vi "walker_tester.vi"() -> ()   [LabVIEW 2010]
uses:
  <userlib>/Nanonis Prog Interface V5/Nanonis Prog Interface.lvlib
panel:
  in  "?":bool
  out "Delta":cluster{"index":i32, sgl}[](graph)
  out "Walk Halt":bool
  out "Walk Done":bool
  in  "Stop Walker":bool
  in  "Stop Loop":bool
  in  "Number of Steps":u16=500
  in  "Capacitance Limit":sgl=700.0
  out "Capacitance":cluster{"index":i32, sgl}[](graph)
  in  "?":bool
  in  "Frequency (Hz)":sgl=250.0
  in  "Amplitude (V)":sgl=150.0
  # "+Z"
  # "-Z"
  # "Absolute Value"
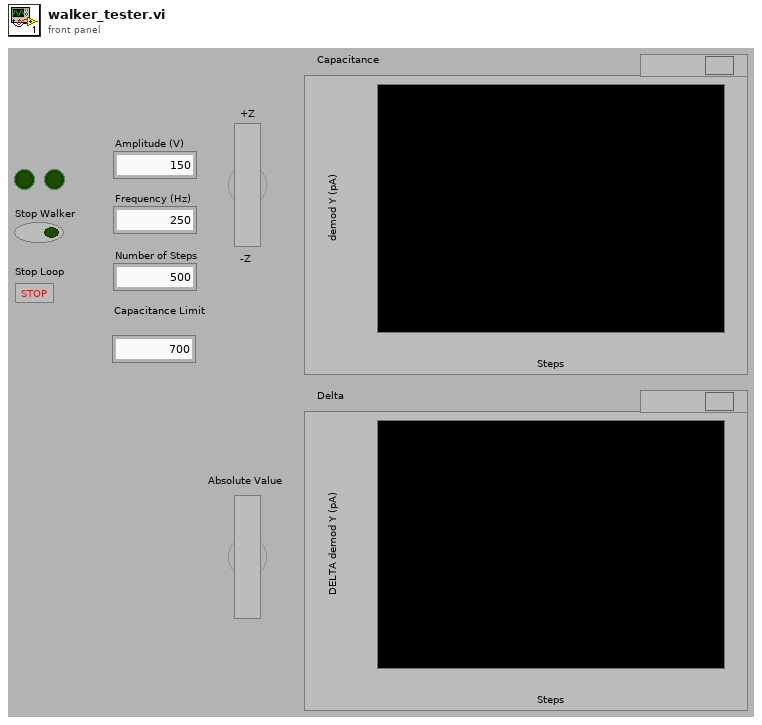
[diagram p1: front panel]
types:
  T1 = enum8{"Group 1", "Group 2", "Group 3", "Group 4", "Group 5", "Group 6"}
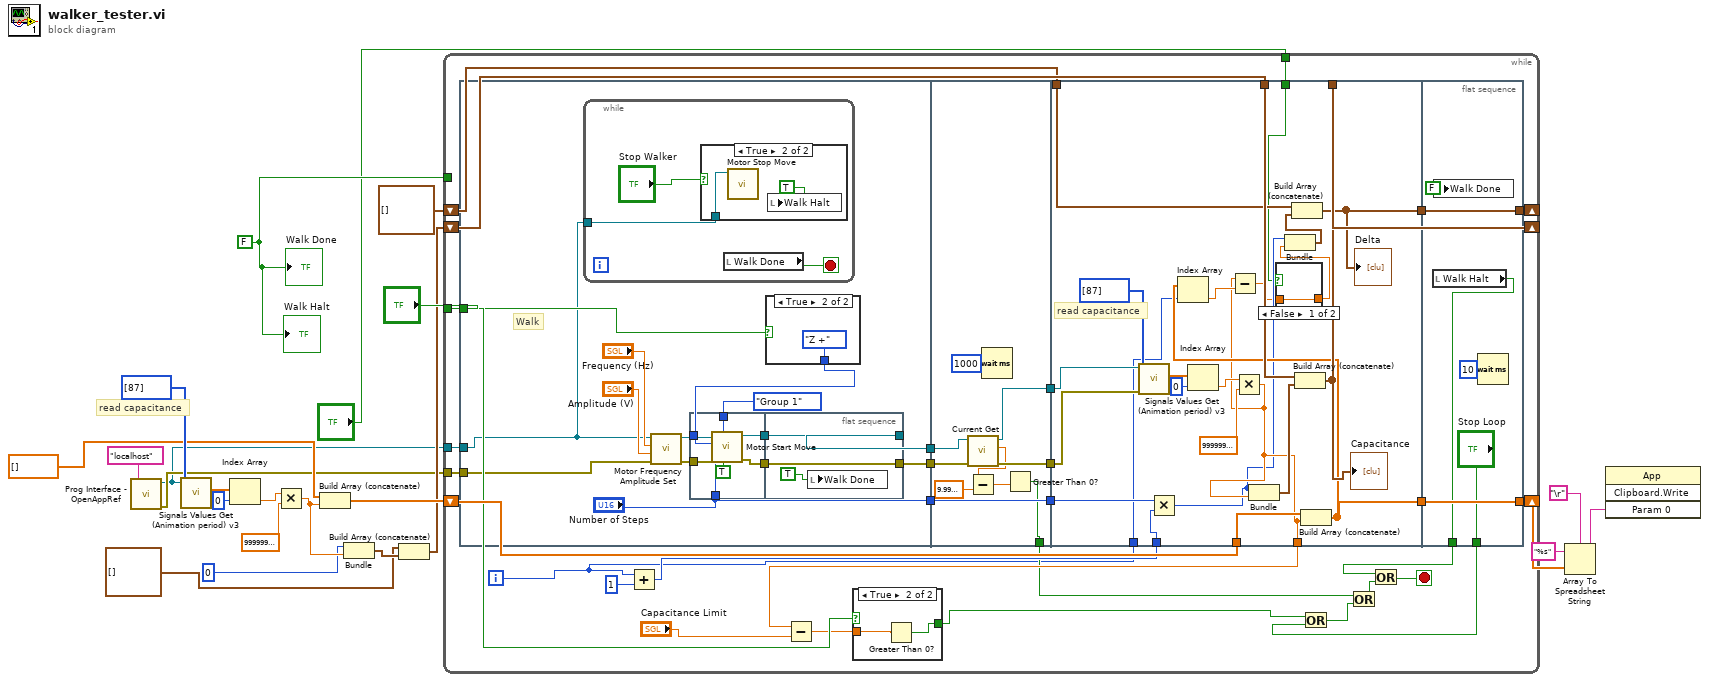
[diagram p0: block diagram]
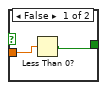
[diagram p2: hidden frame]
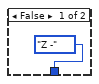
[diagram p4: hidden frame]
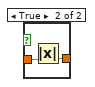
[diagram p5: hidden frame]
diagram:
  w3 = FALSE
  # "read capacitance"
  n1 = call <userlib>:"Prog Interface - OpenAppRef.vi"("Machine name (local machine IP)"="localhost" ("machine name (localhost)")) -> ("Error out"=w5:errorcluster, "Application reference"=w4:refnum<vi>)  [unwired: 5 in]
  n2 = call <userlib>:"Signals Values Get (Animation period) v3.vi"("Signals indexes (0-127)"=i8[] [87], "Application ref in"=w4) -> ("Signals Values"=w15:sgl[])  [unwired: 6 in, 2 out]
  n3 = Index Array(array=w15, index=0) -> (element=w14:sgl)
  n4 = Multiply(x=w14, y=sgl 1000000000000.0) -> (x*y=w10:sgl)
  n5 = Build Array (concatenate)(sgl[] [], w10) -> (w11:sgl[])
  n6 = Bundle("index"=0, w10) -> (w8:cluster{"index":i32, sgl})  [unwired: 1 in]
  n7 = Build Array (concatenate)(cluster{i32, sgl}[] [], w8) -> (w7:cluster{"index":i32, sgl}[])
  n8 = while {
    shift-right: [w52] -> _
    shift-left: w7 -> [w51]
    shift-right: [w50] -> w23
    shift-left: w11 -> [w49]
    tunnel: "?" -> [w47]
    tunnel: w4 -> [w39]
    tunnel: w5 -> [w38]
    tunnel: w3 -> [_]
    shift-right: [w26] -> _
    shift-left: cluster{i32, sgl}[] [] -> [w25]
    tunnel: "?" -> [w24]
    i -> [w28]
    stop <- w31 stop-if-true
    n9 = flat-sequence {
      tunnel: ["Number of Steps"] -> w54
      tunnel: w47 -> [w66]
      tunnel: w39 -> [w61]
      tunnel: w38 -> [w64]
      tunnel: [w63] -> w37
      tunnel: [w62] -> w36
      tunnel: w54 -> [w99]
      tunnel: [w99] -> w53
      tunnel: w37 -> [w98]
      tunnel: w36 -> [w97]
      tunnel: [w96] -> w35
      tunnel: [w95] -> w34
      tunnel: [w92] -> w32
      tunnel: [w117] -> w52
      tunnel: w40 -> [w119]
      tunnel: w53 -> [w114]
      tunnel: w51 -> [w116]
      tunnel: w49 -> [w115]
      tunnel: [w108] -> w48
      tunnel: [w111] -> w43
      tunnel: w35 -> [w113]
      tunnel: w34 -> [w112]
      tunnel: w28 -> [w110]
      tunnel: [w104] -> w27
      tunnel: w25 -> [w105]
      tunnel: w24 -> [w101]
      tunnel: [w133] -> w50
      tunnel: w43 -> [w133]
      tunnel: ["Stop Loop"] -> w42
      tunnel: [w129] -> w29
      tunnel: w27 -> [w128]
      tunnel: [w128] -> w26
      frame #0 {
        # "Walk"
        n10 = while {
          tunnel: w61 -> [w74]
          stop <- w73 stop-if-true
          n11 = case shown="True" "Stop Walker" {
            tunnel: w74 -> [_ w77]
            frame False {
            }
            frame True {
              n12 = call <userlib>:"Motor Stop Move.vi"("Application ref in"=w77) -> ()  [unwired: 9 in, 2 out]
              n13 = local write "Walk Halt"(TRUE ("Wait until finished? (F)")) -> ()
            }
          }
          n14 = local read "Walk Done"() -> (w73:bool)
        }
        n15 = call <userlib>:"Motor Frequency Amplitude Set.vi"("Error in (no error)"=w64, "Amplitude (V) (NaN=no change)"="Amplitude (V)", "Frequency (Hz) (NaN=no change)"="Frequency (Hz)", "Application ref in"=w61) -> ("Error out"=w68:errorcluster, "Application ref out"=w69:refnum<vi>)  [unwired: 6 in]
        n16 = flat-sequence {
          tunnel: T1."Group 1" ("Group") -> [w84]
          tunnel: w69 -> [w83]
          tunnel: w68 -> [w82]
          tunnel: w67 -> [w81]
          tunnel: "Number of Steps" -> [w80]
          tunnel: [w79] -> w60
          tunnel: [w78] -> w59
          tunnel: [w87] -> w62
          tunnel: [w88] -> w63
          tunnel: w60 -> [w88]
          tunnel: w59 -> [w87]
          frame #0 {
            n17 = call <userlib>:"Motor Start Move.vi"("Wait until finished? (F)"=TRUE, "Group"=w84, "Error in (no error)"=w82, "Number of steps"=w80, "Direction"=w81, "Application ref in"=w83) -> ("Error out"=w78:errorcluster, "Application ref out"=w79:refnum<vi>)  [unwired: 3 in]
          }
          frame #1 {
            n18 = local write "Walk Done"(TRUE ("Wait until finished? (F)")) -> ()
          }
        }
        n19 = case shown="True" w66 {
          tunnel: [enum16{"X +", "X -", "Y +", "Y -", "Z +", "Z -"}."Z -" ("Direction") enum16{"X +", "X -", "Y +", "Y -", "Z +", "Z -"}."Z +" ("Direction")] -> w67
          frame False {
          }
          frame True {
          }
        }
      }
      frame #1 {
        n20 = call <userlib>:"Current Get.vi"("Error in (no error)"=w97, "Application ref in"=w98) -> ("Error out"=w96:errorcluster, "Current (A)"=w94:sgl, "Application ref out"=w95:refnum<vi>)  [unwired: 5 in]
        n21 = Subtract(x=w94, y=sgl 1e-09) -> (x-y=w93:sgl)
        n22 = Wait (ms)(milliseconds to wait=u32 1000) -> ()  [unwired: 1 out]
        n23 = Greater Than 0?(x=w93) -> (x > 0?=w92:bool)
      }
      frame #2 {
        # "read capacitance"
        n24 = call <userlib>:"Signals Values Get (Animation period) v3.vi"("error in (no error)"=w113, "Signals indexes (0-127)"=i8[] [87], "Application ref in"=w112) -> ("Signals Values"=w122:sgl[])  [unwired: 5 in, 2 out]
        n25 = Multiply(x=w114, y=w119) -> (x*y=w107:i32)
        n26 = Index Array(array=w122, index=0) -> (element=w121:sgl)
        n27 = Multiply(x=w121, y=sgl 1000000000000.0) -> (x*y=w108:sgl)
        n28 = Bundle(w107, w108) -> (w118:cluster{i32, sgl})  [unwired: 1 in]
        n29 = Build Array (concatenate)(w116, w118) -> (w117:cluster{"index":i32, sgl}[])
        "Capacitance" <- w117
        n30 = Build Array (concatenate)(w115, w108) -> (w111:sgl[])
        n31 = Index Array(array=w111, index=w110) -> (element=w109:sgl)
        n32 = Subtract(x=w108, y=w109) -> (x-y=w103:sgl)
        n33 = case shown="False" w101 {
          tunnel: w103 -> [w125 w127]
          tunnel: [w125 w126] -> w102
          frame False {
          }
          frame True {
            n34 = Absolute Value(x=w127) -> (abs(x)=w126:sgl)
          }
        }
        n35 = Bundle(w107, w102) -> (w106:cluster{i32, sgl})  [unwired: 1 in]
        n36 = Build Array (concatenate)(w105, w106) -> (w104:cluster{i32, sgl}[])
        "Delta" <- w104
      }
      frame #3 {
        n37 = local read "Walk Halt"() -> (w129:bool)
        n38 = local write "Walk Done"(FALSE ("Walker Halt")) -> ()
        n39 = Wait (ms)(milliseconds to wait=u32 10) -> ()  [unwired: 1 out]
      }
    }
    n40 = Add(x=w28, y=u16 1) -> (x+y=w40:i32)
    n41 = Subtract(x=w48, y="Capacitance Limit") -> (x-y=w45:sgl)
    n42 = case shown="True" w47 {
      tunnel: w45 -> [w55 w58]
      tunnel: [w56 w57] -> w44
      frame False {
        n43 = Less Than 0?(x=w55) -> (x < 0?=w56:bool)
      }
      frame True {
        n44 = Greater Than 0?(x=w58) -> (x > 0?=w57:bool)
      }
    }
    n45 = Or(x=w44, y=w42) -> (x .or. y?=w33:bool)
    n46 = Or(x=w32, y=w33) -> (x .or. y?=w30:bool)
    n47 = Or(x=w29, y=w30) -> (x .or. y?=w31:bool)
  }
  n48 = Array To Spreadsheet String(delimiter (Tab)="\r", array=w23, 3:"%s" ("format string")) -> (spreadsheet string=w22:string)
  n49 = invoke class="App" method="Clipboard.Write"("Param 0"=w22) -> ()  [unwired: 3 in, 4 out]
  "Walk Done" <- w3
  "Walk Halt" <- w3
